vi "xy_bar_graph.vi"() -> ()   [LabVIEW 2014]
doc: "This VI demonstrates how to create a bar graph in LabVIEW by plotting data to an XY graph. This VI converts the data that appears in a table to bars and groups the bars by column of data from the table."
panel:
  out "Annual Report":cluster{dbl[], dbl[]}[](graph)
  in  "Table":string[][](table)=[["34", "74", "23", "35", "23", "26", "74", "74", "21", "39", "61", "83"], ["73", "24", "75", "87", "42", "34", "35", "76", "52", "43", "43", "3"], ["36", "25", "12", "34", "24", "74", "73", "54", "88", "64", "90", "62"]]
  # "This VI graphs the data from the Table to the Annual Report graph.  Select Help»Show Context Help and move the cursor over the VI icon to display help for this VI."
  # "Jan"
  # "Feb"
  # "Mar"
  # "April"
  # "May"
  # "June"
  # "July"
  # "Aug"
  # "Sept"
  # "Oct"
  # "Nov"
  # "Dec"
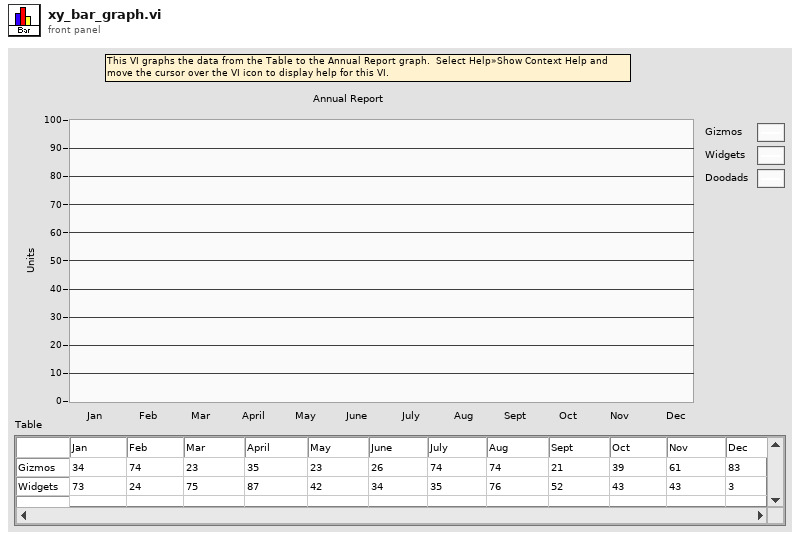
[diagram p1: front panel]
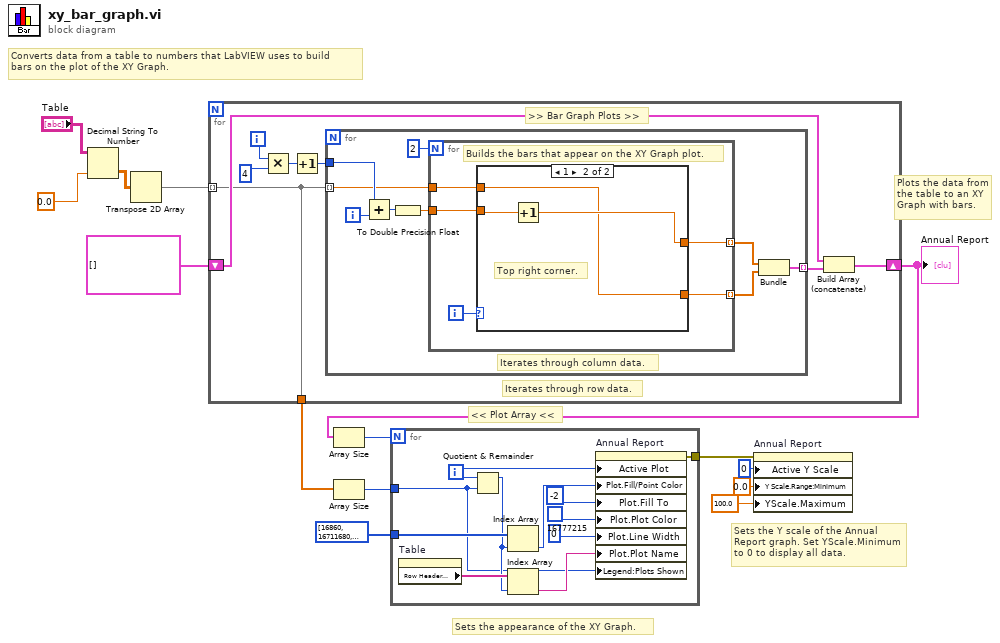
[diagram p0: block diagram]
diagram:
  # "Plots the data from the table to an XY Graph with bars."
  # "Converts data from a table to numbers that LabVIEW uses to build \nbars on the plot of the XY Graph."
  # "Sets the appearance of the XY Graph."
  # "Sets the Y scale of the Annual Report graph. Set YScale.Minimum to 0 to display all data."
  # "<< Plot Array <<"
  n1 = Decimal String To Number(string="Table", default (0L)=0.0) -> (number=w12:dbl[][])  [unwired: 2 out]
  n2 = Transpose 2D Array(2D array=w12) -> (transposed array=w11:dbl[][])
  n3 = for {
    tunnel: w11 -> [w15] mode=indexing
    shift-right: [w19] -> w9
    shift-left: cluster{dbl[], dbl[]}[] [] -> [w18]
    tunnel: [w15] -> w7
    i -> [w22]
    # "Iterates through row data."
    # ">> Bar Graph Plots >>"
    n4 = Multiply(x=w22, y=4) -> (x*y=w17:i32)
    n5 = Increment(x=w17) -> (x+1=w16:i32)
    n6 = for {
      tunnel: w15 -> [w24] mode=indexing
      tunnel: w16 -> [w31]
      tunnel: [w26] -> w20 mode=indexing
      i -> [w25]
      # "Iterates through column data."
      n7 = Add(x=w31, y=w25) -> (x+y=w30:i32)
      n8 = To Double Precision Float(number=w30) -> (double precision float=w29:dbl)
      n9 = for {
        N: 2 -> [_]
        tunnel: w24 -> [w35]
        tunnel: [w34] -> w27 mode=indexing
        tunnel: w29 -> [w33]
        tunnel: [w32] -> w28 mode=indexing
        i -> [w36]
        # "Builds the bars that appear on the XY Graph plot."
        n10 = case shown="1" w36 {
          tunnel: w35 -> [w38 w39]
          tunnel: [w38 w39] -> w34
          tunnel: w33 -> [w37 w41]
          tunnel: [w37 w40] -> w32
          frame 0, Default {
            # "Top left corner."
          }
          frame 1 {
            # "Top right corner."
            n11 = Increment(x=w41) -> (x+1=w40:dbl)
          }
        }
      }
      n12 = Bundle(w28, w27) -> (w26:cluster{dbl[], dbl[]})  [unwired: 1 out]
    }
    n13 = Build Array (concatenate) "Build Array"(w18, w20) -> (w19:cluster{dbl[], dbl[]}[])
  }
  "Annual Report" <- w9
  n14 = Array Size(array=w9) -> (size(s)=w8:i32)
  n15 = Array Size(array=w7) -> (size(s)=w6:i32)
  n16 = for {
    N: w8 -> [_]
    tunnel: w6 -> [w43]
    tunnel: u32[] [16860, 16711680, 1175296, 16773632, 15679744, 16711925, 2818015, 4325415] -> [w48]
    tunnel: [w42] -> w4
    i -> [w52]
    n17 = property on="Table" class="Tbl (strict)"() -> ("Row Header Strings[]"=w46:string[])  [unwired: 2 in, 2 out]
    n18 = Quotient & Remainder(x=w52, y=w43) -> (x-y*floor(x/y)=w45:i32)  [unwired: 1 out]
    n19 = Index Array(array=w48, index=w45) -> (element=w51:u32)
    n20 = Index Array(array=w46, index=w45) -> (element=w44:string)
    n21 = property on="Annual Report" class="XYGraph (strict)"("Active Plot"=w52, "Plot.Fill/Point Color"=w51, "Plot.Fill To"=i16 -2, "Plot.Plot Color"=u32 16777215, "Plot.Line Width"=u8 0, "Plot.Plot Name"=w44, "Legend:Plots Shown"=w43) -> (error out=w42:errorcluster)  [unwired: 2 in, 1 out]
  }
  n22 = property on="Annual Report" class="XYGraph (strict)"(error in=w4, "Active Y Scale"=0 ("Active X Scale"), "Y Scale.Range:Minimum"=0.0 ("X Scale.Range:Maximum"), "YScale.Maximum"=100.0 ("Y Scale.Range:Maximum")) -> ()  [unwired: 1 in, 2 out]
